vi "setRootDevice.vi"(8 "error in (no error)":errorcluster, 9 "Config in":refnum<class "IPropertyObject.lvclass">, 10 "RootDeviceName":string, 11 "IInstanceBuilder in":refnum<class "IInstanceBuilder.lvclass">) -> (0 "error out":errorcluster, 1 "Config out":refnum<class "IPropertyObject.lvclass">, 3 "IInstanceBuilder out":refnum<class "IInstanceBuilder.lvclass">)   [LabVIEW 2022 SP3, in "openDAQ.lvlib" / "IBaseObject.lvlib" / "IInstanceBuilder.lvlib" / "IInstanceBuilder.lvclass"]
uses:
  <instrlib>/openDAQ/Public/Classes/IInstanceBuilder/IInstanceBuilder.lvclass
  <instrlib>/openDAQ/Public/Classes/IInstanceBuilder/IInstanceBuilder.lvclass/IInstanceBuilder.ctl
  <instrlib>/openDAQ/Public/Classes/daqCoreTypes/IString/IString.lvclass
  <instrlib>/openDAQ/Binaries/Windows/x86/copendaq32.dll
  <instrlib>/openDAQ/Public/Classes/IPropertyObject/IPropertyObject.lvclass
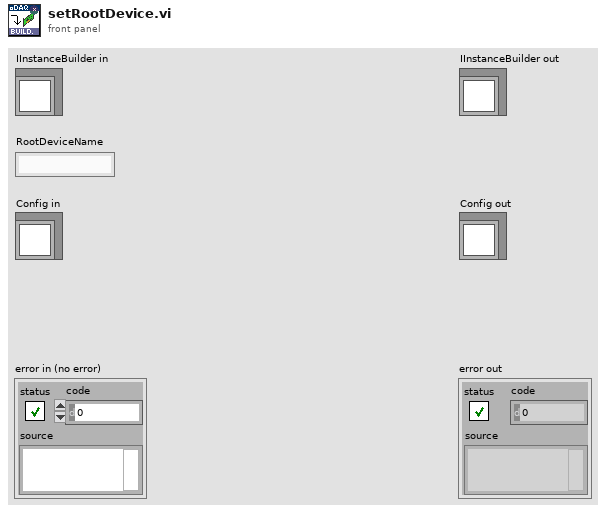
[diagram p1: front panel]
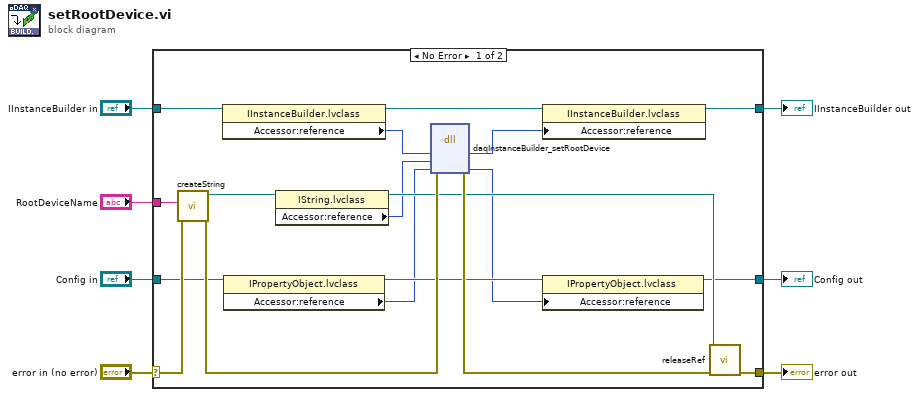
[diagram p0: block diagram]
diagram:
  n1 = case shown="No Error" "error in (no error)" {
    selector: "error in (no error)" -> [w24 w28]
    tunnel: [w16 w28] -> w6
    tunnel: [w18 w27] -> w4
    tunnel: "IInstanceBuilder in" -> [w19 w27]
    tunnel: "RootDeviceName" -> [w25 _]
    tunnel: "Config in" -> [w13 w26]
    tunnel: [w10 w26] -> w1
    frame No Error {
      n2 = call <instrlib>:"createString.vi"("error in (no error)"=w24, "String"=w25) -> ("error out"=w22:errorcluster, "IString out"=w21:refnum<class "IString.lvclass">)  [unwired: 8 in]
      n3 = property class="IInstanceBuilder.lvclass"(reference=w19) -> (reference out=w17:refnum<class "IInstanceBuilder.lvclass">, "Accessor:reference"=w15:i64)  [unwired: 1 in, 1 out]
      n4 = property class="IPropertyObject.lvclass"(reference=w13) -> (reference out=w12:refnum<class "IPropertyObject.lvclass">, "Accessor:reference"=w11:i64)  [unwired: 1 in, 1 out]
      n5 = property class="IString.lvclass"(reference=w21) -> (reference out=w20:refnum<class "IString.lvclass">, "Accessor:reference"=w14:i64)  [unwired: 1 in, 1 out]
      n6 = dll-call lib="C:/Program Files (x86)/National Instruments/LabVIEW 2022/instr.lib/openDAQ/Binaries/Windows/x86/copendaq*.*" fn="daqInstanceBuilder_setRootDevice"(error in=w22, "instanceBuilder"=w15, "rootDeviceName"=w14, "config"=w11) -> (error out=w23:errorcluster, "instanceBuilder"=w8:i64, "config"=w9:i64)  [unwired: 4 in, 1 out]
      n7 = property class="IInstanceBuilder.lvclass"(reference=w17, "Accessor:reference"=w8) -> (reference out=w18:refnum<class "IInstanceBuilder.lvclass">)  [unwired: 1 in, 1 out]
      n8 = property class="IPropertyObject.lvclass"(reference=w12, "Accessor:reference"=w9) -> (reference out=w10:refnum<class "IPropertyObject.lvclass">)  [unwired: 1 in, 1 out]
      n9 = call-dynamic "releaseRef.vi"("error in (no error)"=w23, "IBaseObject in"=w20) -> ("error out"=w16:errorcluster)  [unwired: 9 in]
    }
    frame Error {
    }
  }
  "error out" <- w6
  "IInstanceBuilder out" <- w4
  "Config out" <- w1
